vi "Save.vi"(8 "error in (no error)":errorcluster, 11 "AB_UI_Fmwrk_Build in":refnum<class "AB_UI_Frmwk_Build.lvclass">) -> (0 "error out":errorcluster, 2 "build spec name":string, 3 "AB_UI_Fmwrk_Build out":refnum<class "AB_UI_Frmwk_Build.lvclass">)   [LabVIEW 2020, in "AB_UI_Frmwk_Build.lvclass"]
uses:
  <vilib>/AppBuilder/AB_Classes/Build/UI/AB_UI_Frmwk_Build.lvclass
  <vilib>/AppBuilder/AB_Classes/Build/AB_Build.lvclass
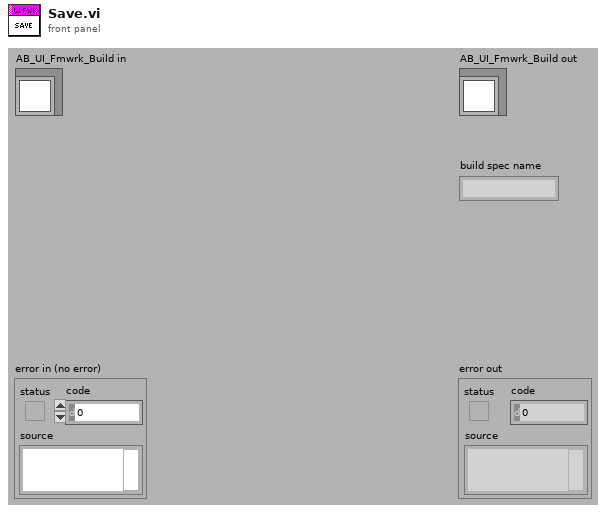
[diagram p1: front panel]
types:
  T1 = typedef "AB_Build.ctl" = cluster{"buildSpecName":string, "buildSpecDescription":string, "destinations":refnum<class "AB_Destination.lvclass">[], "exclusionOption":T2, "defaultLanguage":string, "supportedLanguages":string[], "excludedDirectories":path[], "buildContext":refnum<vi>, "buildObject":T3, "preview":bool, "programatic":bool, "progressBarEvents":T4, "userLog_Path":path, "preActionID":string, "preAction_Path":path, "postActionID":string, "postAction_Path":path, "eng_checkForBrokenVIs?":bool, "eng_verboseLinkerErrors?":bool, "localDest_Path":path, "targetDest_Path":path, "removeVIObject":u16, "cache":refnum<class "PreviewCache.lvclass">, "use cache":bool, "previewCache_ID":string, "buildCache_ID":string, "eng_TempLocalDest_Path":path, "eng_collectDependencies?":bool, "versionInfo":cluster{"buildVersion":cluster{"major":u16, "minor":u16, "patch":u16, "build":u16}, "autoIncrement":bool}, "eng_enableVIChecksums":bool}
  T2 = typedef "AB_Exclusion_Option.ctl" = cluster{"typedefs":bool, "polymorphicVIs":bool, "unusedLibraryItems":bool, "modifyLibraryFile":bool, "edit-timeDependencies":bool, "inlineVIs":bool, "dependent PPLs":bool, "dependent DLLs":bool}
  T3 = typedef "ItemRef.ctl" = u64
  T4 = typedef "provcom_ProgressBar_Events.ctl" = cluster{"newJob":refnum<user-event>, "newItem":refnum<user-event>, "errorMsg":T5, "cancel":refnum<user-event>}
  T5 = typedef "mxLvBuildError.ctl" = refnum<user-event>
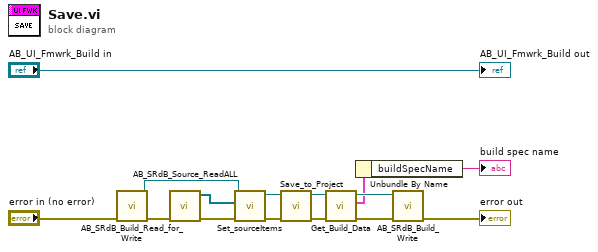
[diagram p0: block diagram]
diagram:
  n1 = call <resource>:"AB_SRdB_Build_Read_for_Write.vi"("error in (no error)"="error in (no error)") -> ("error out"=w9:errorcluster, "build out"=w10:refnum<class "AB_Build.lvclass">)  [unwired: 9 out]
  n2 = call <resource>:"AB_SRdB_Source_ReadALL.vi"("error in (no error)"=w9) -> ("error out"=w8:errorcluster, "ALL data"=w7:refnum<class "AB_Source.lvclass">[])  [unwired: 9 out]
  n3 = call <vilib>:"Set_sourceItems.vi"("error in (no error)"=w8, "sourceItems"=w7, "Class in"=w10) -> ("error out"=w6:errorcluster, "Class out"=w5:refnum<class "AB_Build.lvclass">)  [unwired: 7 out]
  n4 = call-dynamic "Save_to_Project.vi"("error in (no error)"=w6, "AB_Build in"=w5) -> ("error out"=w14:errorcluster, "AB_Build out"=w12:refnum<class "AB_Build.lvclass">)  [unwired: 8 out]
  n5 = call <vilib>:"Get_Build_Data.vi"("error in (no error)"=w14, "Class in"=w12) -> ("error out"=w15:errorcluster, "data"=w11:T1, "Class out"=w13:refnum<class "AB_Build.lvclass">)  [unwired: 7 out]
  n6 = Unbundle By Name(w11) -> ("buildSpecName"=→"build spec name":string)
  n7 = call <resource>:"AB_SRdB_Build_Write.vi"("error in (no error)"=w15, "build in"=w13) -> ("error out"=→"error out":errorcluster)  [unwired: 9 out]
  "AB_UI_Fmwrk_Build out" <- "AB_UI_Fmwrk_Build in"
